vi "Load Animation.vi"(8 "Error In":errorcluster, 9 "Position":cluster{"X":i16, "Y":i16}, 10 "FPS":u32=30, 11 "Animation Picture Indicator":refnum<vi>) -> (0 "Error Out":errorcluster, 3 "Animation Config":T1)   [LabVIEW 2011, in "LVH-Toolbox.lvlib" / "GUI Tools.lvlib"]
uses:
  GUI Tools.lvlib
  Private/Animations/Type Defs/Animation Config.ctl
  <vilib>/picture/picture.llb/imagedata.ctl
  Private/Animations/FGVs/Type Defs/Animation FGV State.ctl
panel:
  out "call chain":string[](array[string])
  in  "Animation":enum16{"Green Bars"}(ring)
  in  "Animation Config":T1
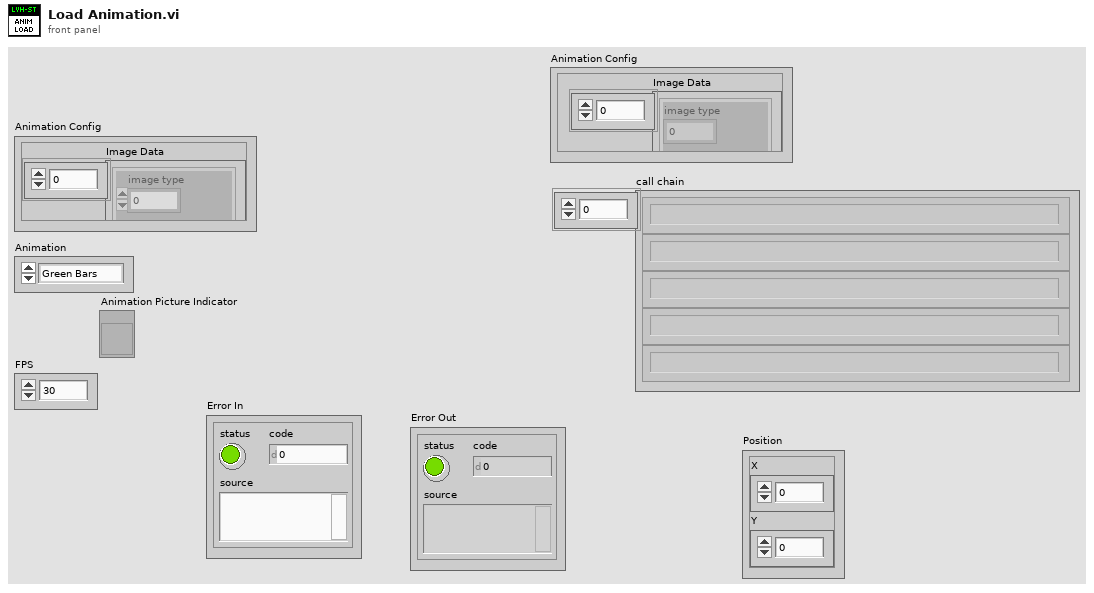
[diagram p1: front panel]
types:
  T1 = typedef "LVH-Toolbox.lvlib/GUI Tools.lvlib/Animation Config.ctl" = cluster{"Image Data":T2[], "Animation Picture Indicator":refnum<vi>, "FPS":u32, "Position":cluster{"X":i16, "Y":i16}}
  T2 = typedef "imagedata.ctl" = cluster{"image type":i32, "image depth":i32, "image":u8[], "mask":u8[], "colors":u32[], "Rectangle":cluster{"left":i16, "top":i16, "right":i16, "bottom":i16}}
  T3 = typedef "LVH-Toolbox.lvlib/GUI Tools.lvlib/Animation FGV State.ctl" = enum16{"Init", "Set", "Get"}
  T4 = typedef "LVRectTypeDef.ctl" = cluster{"left":i16, "top":i16, "right":i16, "bottom":i16}
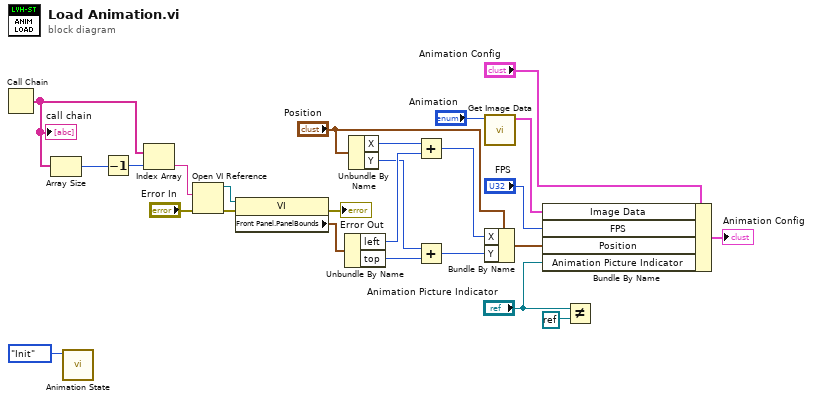
[diagram p0: block diagram]
diagram:
  n1 = Call Chain() -> (call chain=w17:string[])
  "call chain" <- w17
  n2 = Array Size(array=w17) -> (size(s)=w19:i32)
  n3 = call "Animation State.vi"("Function"=Animation_FGV_State."Init") -> ()  [unwired: 10 in, 1 out]
  n4 = Decrement(x=w19) -> (x-1=w18:i32)
  n5 = Index Array(array=w17, index=w18) -> (element=w16:string)
  n6 = Open VI Reference(vi path=w16, error in (no error)="Error In") -> (vi reference=w15:refnum<vi>, error out=w14:errorcluster)  [unwired: 4 in]
  n7 = property class="VI"(reference=w15, error in=w14) -> (error out=→"Error Out":errorcluster, "Front Panel.PanelBounds"=w13:T4)  [unwired: 1 out]
  n8 = Unbundle By Name(w13) -> ("left"=w11:i16, "top"=w9:i16)
  n9 = Unbundle By Name("Position") -> ("X"=w12:i16, "Y"=w10:i16)
  n10 = Add(x=w12, y=w11) -> (x+y=w8:i16)
  n11 = Add(x=w10, y=w9) -> (x+y=w7:i16)
  n12 = call "Get Image Data.vi"("Animation"="Animation") -> ("Frame Data"=w20:T2[])  [unwired: 10 in]
  n13 = Bundle By Name(cluster="Position", "X"=w8, "Y"=w7) -> (w5:cluster{"X":i16, "Y":i16})
  n14 = Bundle By Name(cluster="Animation Config", "Image Data"=w20, "FPS"="FPS", "Position"=w5, "Animation Picture Indicator"="Animation Picture Indicator") -> (→"Animation Config":T1)
  n15 = Not Equal?(x="Animation Picture Indicator", y=refnum<k0> refnum) -> ()  [unwired: 1 out]
